vi "Flush Log.vi"(8 "error in (no error)":errorcluster, 11 "CoolAppProcess in":refnum<class "CoolAppProcess.lvclass">) -> (0 "error out":errorcluster, 2 "remaining elements":string[](array[string]), 3 "CoolAppProcess out":refnum<class "CoolAppProcess.lvclass">)   [LabVIEW 2020, in "LAF2024Q2.lvlib" / "CoolAppProcess.lvclass"]
uses:
  CoolAppProcess.lvclass
  CoolAppProcess.lvclass/CoolAppProcess.ctl
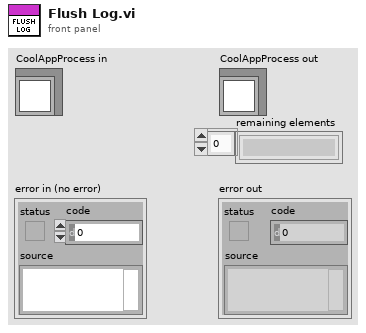
[diagram p1: front panel]
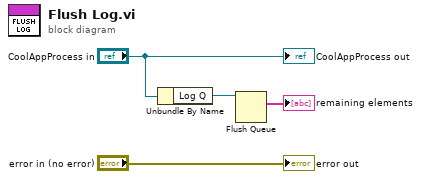
[diagram p0: block diagram]
diagram:
  n1 = Unbundle By Name("CoolAppProcess in") -> ("Log Q"=w2:refnum<queue>)
  n2 = Flush Queue(queue=w2) -> (remaining elements=→"remaining elements":string[])  [unwired: 1 in, 2 out]
  "error out" <- "error in (no error)"
  "CoolAppProcess out" <- "CoolAppProcess in"
